vi "FPGA_SPI_StartAuto_Timed.vi"(8 "error in (no error)":errorcluster, 11 "Sample Period (us)":u32) -> (0 "error out":errorcluster)   [LabVIEW 2017]
uses:
  <vilib>/Utility/error.llb/Error Cluster From Error Code.vi
  <vilib>/rvi/errors/niLvFpgaAdjustHostInterfaceError.vi
  <vilib>/rvi/interface/nirviReadWriteControl/nirviReadWriteControl.xnode
  <vilib>/Rock Robotics/SystemInterfaces/System/FPGA_SystemFRC FPGA Ref.ctl
  <vilib>/rvi/interface/Simulation/niFpgaSimulationCallBeginRW.vi
  NiFpgaLv.dll
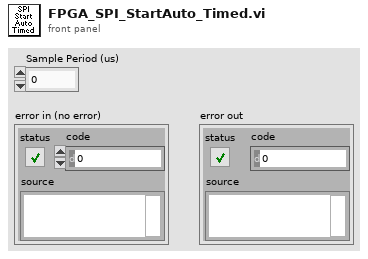
[diagram p1: front panel]
types:
  T1 = typedef "FPGA_SystemFRC FPGA Ref.ctl" = refnum<k20>
  T2 = cluster{"ExternalClockSource":cluster{"Channel":fxp<+,4,4>, "Module":fxp<+,1,1>, "AnalogTrigger":bool}, "RisingEdge":bool, "FallingEdge":bool, "ExternalClock":bool}
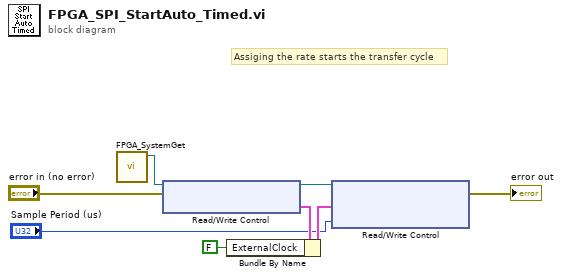
[diagram p0: block diagram]
diagram:
  # "Assiging the rate starts the transfer cycle"
  n1 = call <vilib>:"FPGA_SystemGet.vi"() -> ("FRC FPGA Ref"=w1:T1)  [unwired: 11 in]
  n2 = xnode "Read/Write Control"("FPGA VI Reference In"=w1, "error in"="error in (no error)") -> ("FPGA VI Reference Out"=w7:T1, "SPI.AutoTriggerConfig"=w6:T2)  [unwired: 1 out]
  n3 = Bundle By Name(cluster=w6, "ExternalClock"=FALSE) -> (w5:T2)
  n4 = xnode "Read/Write Control"("FPGA VI Reference In"=w7, "SPI.AutoTriggerConfig"=w5, "SPI.AutoRate"="Sample Period (us)") -> ("error out"=→"error out":errorcluster)  [unwired: 1 in, 1 out]
